vi "例4.16 局部变量输出循环结构内的数据2.vi"() -> ()   [LabVIEW 2017]
panel:
  in  "停止":bool
  out "Y":dbl
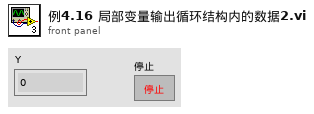
[diagram p1: front panel]
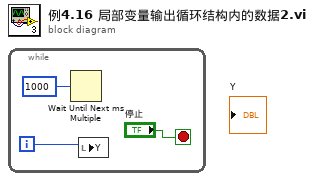
[diagram p0: block diagram]
diagram:
  n1 = while {
    i -> [w2]
    stop <- "停止" stop-if-true
    n2 = Wait Until Next ms Multiple(millisecond multiple=u32 1000 ("毫秒倍数")) -> ()  [unwired: 1 out]
    n3 = local write "Y"(w2) -> ()
  }
